vi "ep_Power Calculation.vi"(9 "Q":dbl, 11 "P":dbl) -> (3 "power values":T1)   [LabVIEW 2013, in "NI_EP_Power Measurement.lvlib"]
uses:
  <vilib>/addons/Electrical Power/Power Measurement/NI_EP_Power Measurement.lvlib
  <vilib>/addons/Electrical Power/Basic/Measurement/subVIs/basic_Power Value.ctl
  <vilib>/addons/Electrical Power/Basic/NI_EP_Basic.lvlib
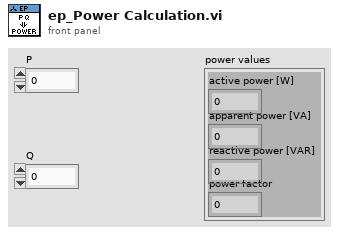
[diagram p1: front panel]
types:
  T1 = typedef "NI_EP_Basic.lvlib/basic_Power Value.ctl" = cluster{"active power [W]":dbl, "apparent power [VA]":dbl, "reactive power [VAR]":dbl, "power factor":dbl}
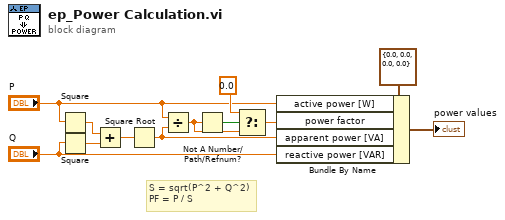
[diagram p0: block diagram]
diagram:
  # "S = sqrt(P^2 + Q^2)\nPF = P / S"
  n1 = Square(x="P") -> (x^2=w9:dbl)
  n2 = Square(x="Q") -> (x^2=w12:dbl)
  n3 = Add(x=w9, y=w12) -> (x+y=w11:dbl)
  n4 = Square Root(x=w11) -> (sqrt(x)=w8:dbl)
  n5 = Divide(x="P", y=w8) -> (x/y=w6:dbl)
  n6 = Not A Number/Path/Refnum?(number/path/refnum=w6) -> (NaN/Path/Refnum?=w7:bool)
  n7 = Select(t=0.0, s=w7, f=w6) -> (s? t:f=w2:dbl)
  n8 = Bundle By Name(cluster=T1 {"active power [W]"=0.0, "apparent power [VA]"=0.0, "reactive power [VAR]"=0.0, "power factor"=0.0} ("total power values"), "active power [W]"="P", "power factor"=w2, "apparent power [VA]"=w8, "reactive power [VAR]"="Q") -> (→"power values":T1)
